vi "Install NIPKG By Name.vi"(0 "Feed directory":path, 5 "Package Name":string, 11 "error in":errorcluster) -> (4 "standard output":string, 15 "error out":errorcluster)   [LabVIEW 2020]
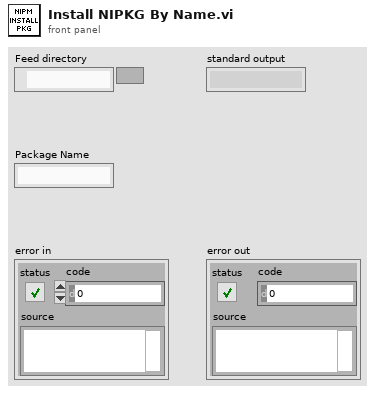
[diagram p1: front panel]
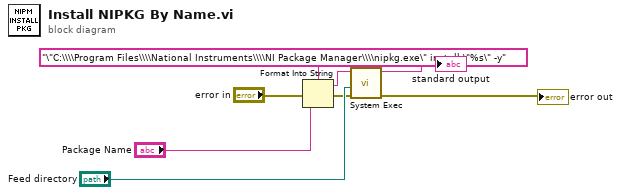
[diagram p0: block diagram]
diagram:
  n1 = Format Into String(format string="\"C:\\\\Program Files\\\\National Instruments\\\\NI Package Manager\\\\nipkg.exe\" install \"%s\" -y" ("command line"), error in="error in", "Package Name") -> (resulting string=w4:string, error out=w3:errorcluster)  [unwired: 1 in]
  n2 = call <vilib>:"System Exec.vi"("error in (no error)"=w3, "working directory"="Feed directory", "command line"=w4) -> ("error out"=→"error out":errorcluster, "standard output"=→"standard output":string)  [unwired: 5 in, 2 out]
